vi "teste_corrente_2LEM.vi"() -> ()   [LabVIEW 2019]
uses:
  <vilib>/Analysis/5stat.llb/RMS (DBL).vi
  <vilib>/Analysis/NI_AALPro.lvlib
  <vilib>/Waveform/WDTFileIO.llb/ Write Waveforms to File (1D).vi
panel:
  in  "Nome de Base do Arquivo - Geral":string="medicoesGerais"
  out "Sucção [ºC]":dbl
  out "Reservatório [ºC]":dbl
  out "Descarga [ºC]":dbl
  out "Corpo [ºC]":dbl
  out "XY Graph 2":cluster{dbl[], dbl[]}[](graph)
  out "Corrente 2 RMS [A]":dbl
  out "Waveform Graph":dynamicdata(graph)
  out "Waveform Chart":dbl[][](graph)
  in  "stop":bool
  out "Corrente RMS [A]":dbl
  in  "Nome de Base do Arquivo - Corrente":string="corr"
  out "Erro Corrente":errorcluster
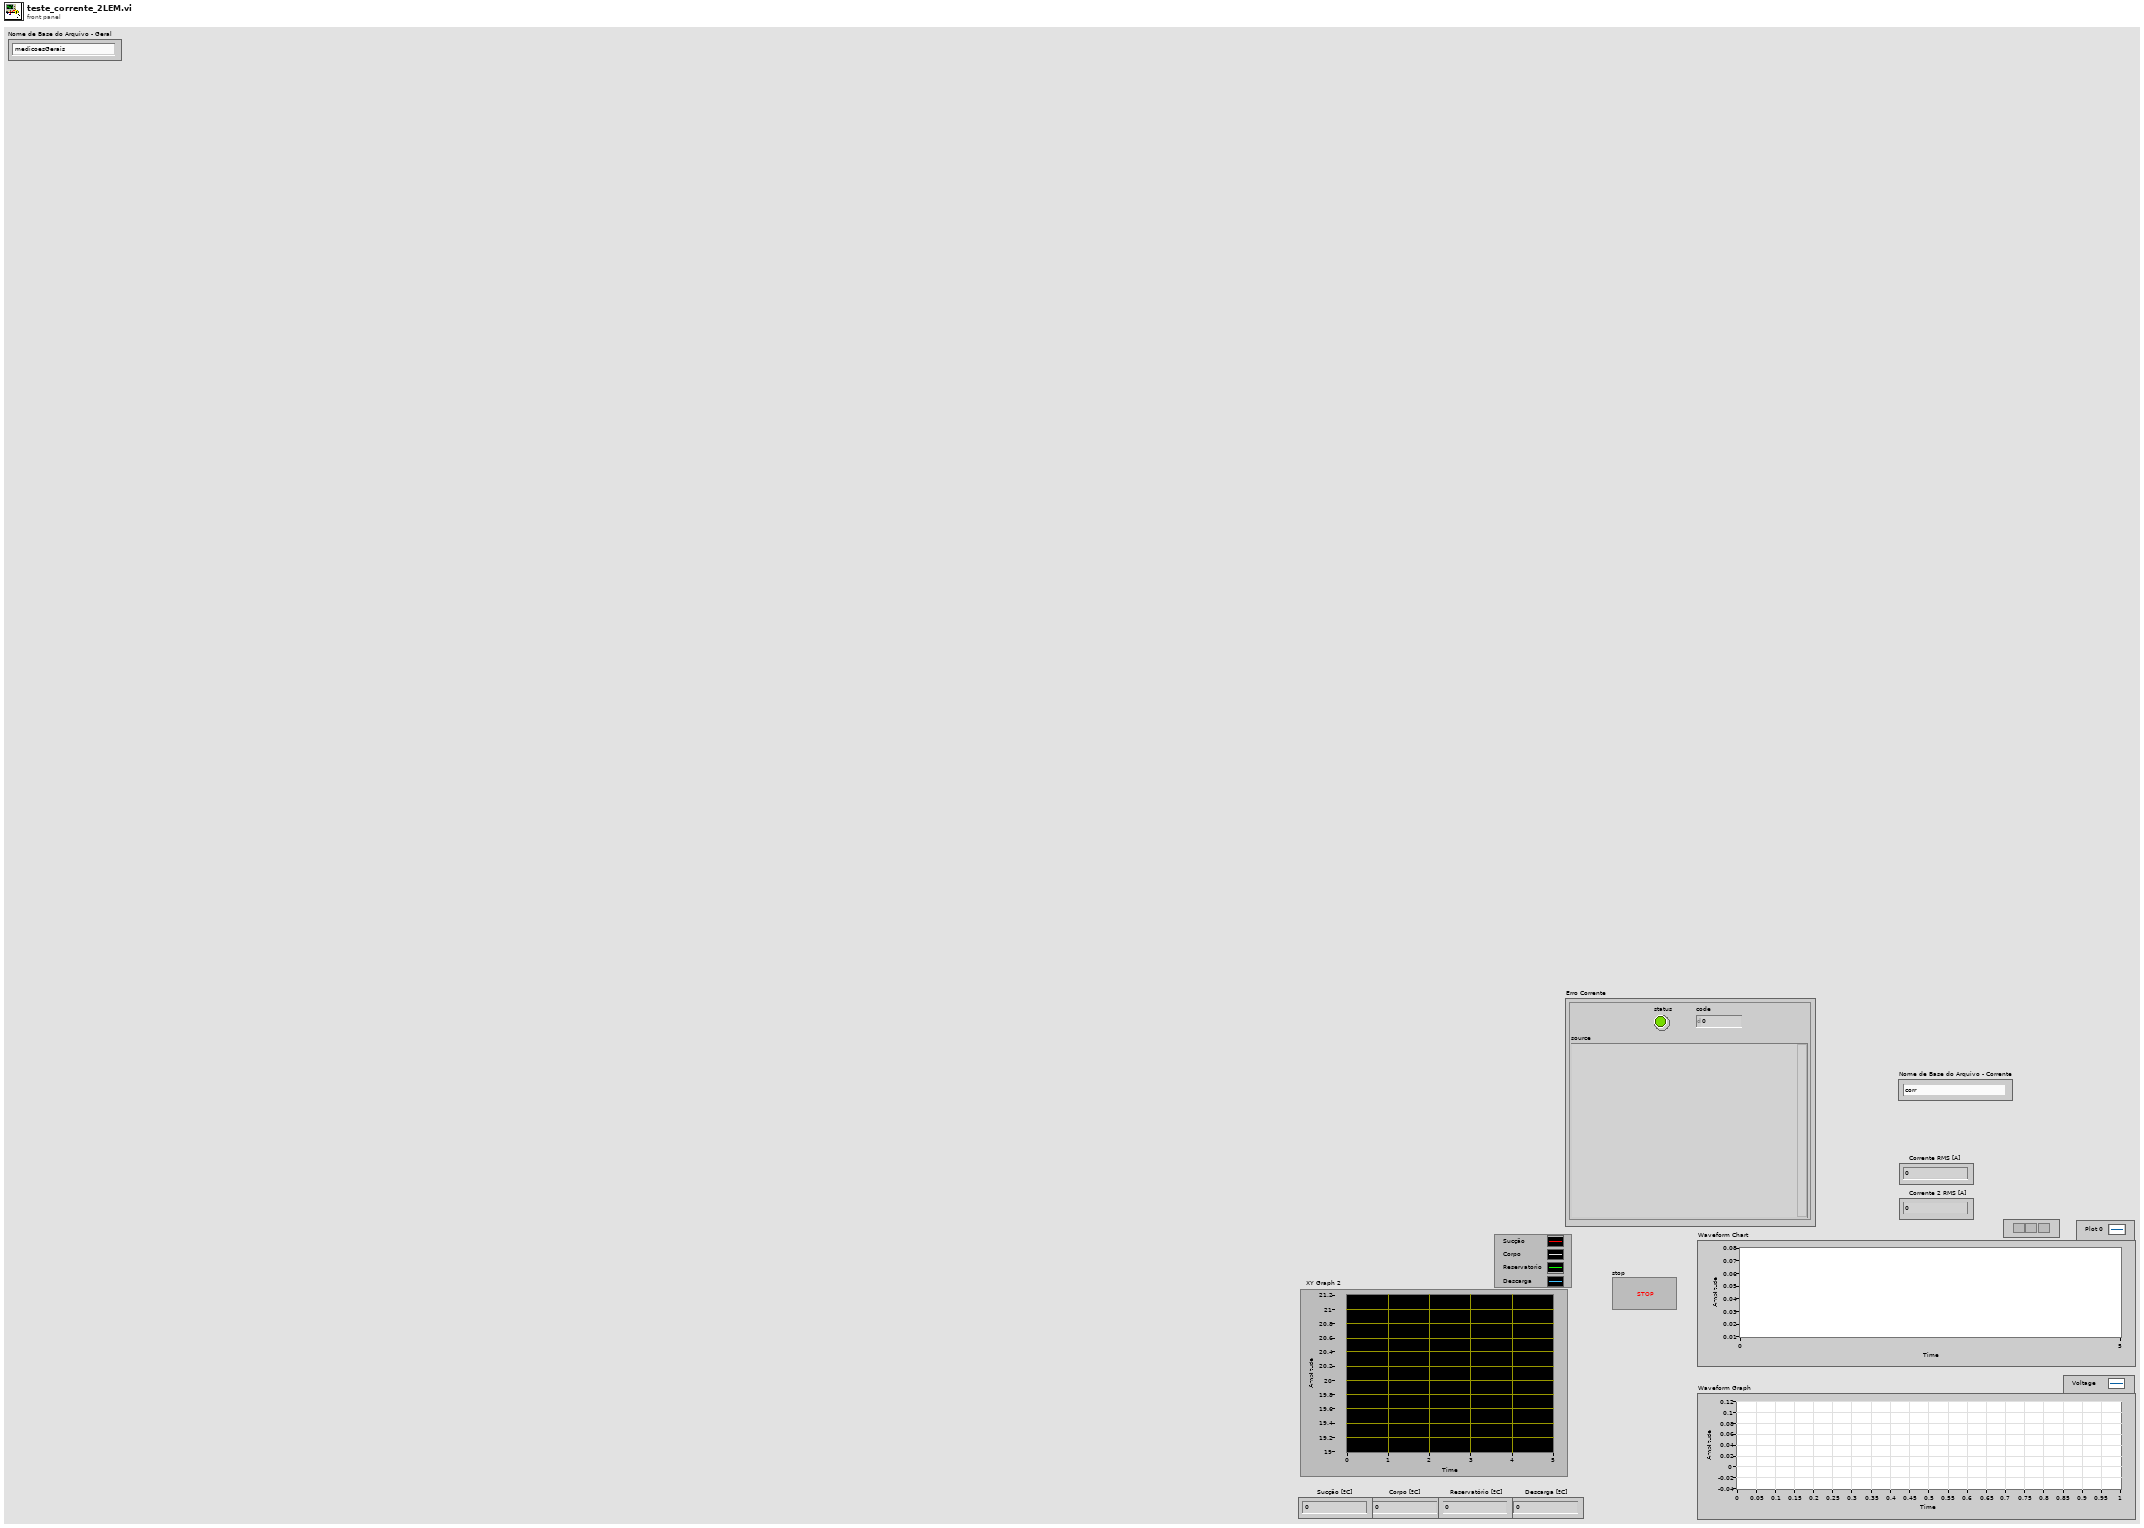
[diagram p1: front panel]
types:
  T1 = enum16{"open", "replace", "create", "open or create", "replace or create", "replace or create with confirmation"}
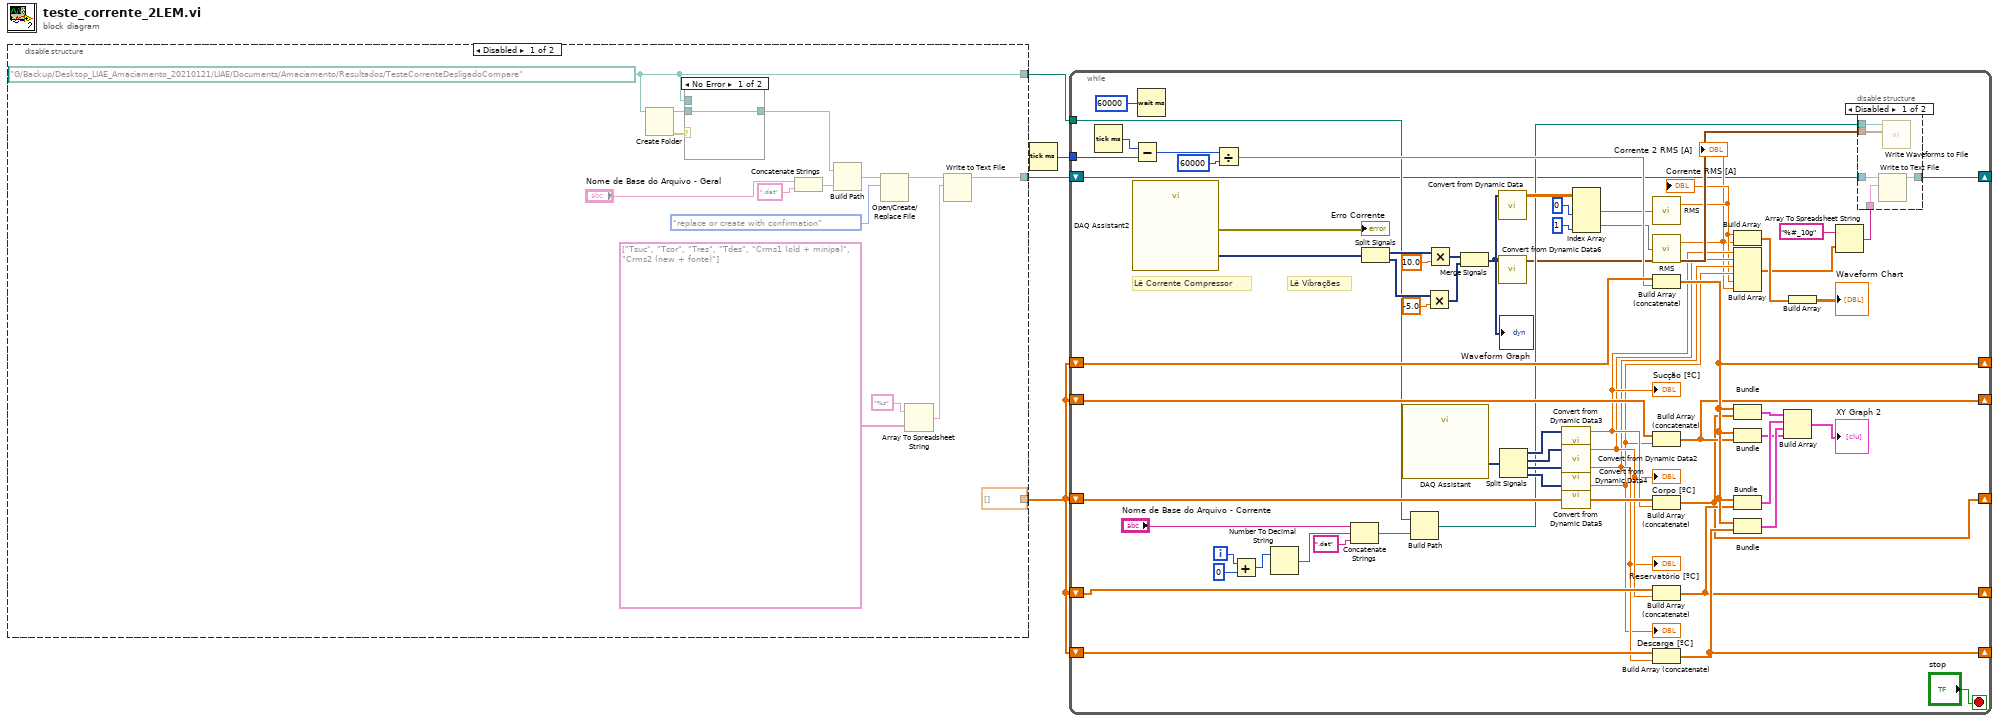
[diagram p0: block diagram]
diagram:
  n1 = disable-structure shown="Disabled" {
    disable-tunnel: [dbl[] [] _] -> w3
    disable-tunnel: [w6 _] -> w2
    disable-tunnel: [w5 _] -> w1
    frame Disabled {
      w5 = path "G:/Backup/Desktop_LIAE_Amaciamento_20210121/LIAE/Documents/Amaciamento/Resultados/TesteCorrenteDesligadoCompare" ("base path")
      n2 = Create Folder(path (use dialog)=w5) -> (created path=w10:path, error out=w11:errorcluster)  [unwired: 2 in, 1 out]
      n3 = case shown="No Error" w11 {
        tunnel: w10 -> [w20 _]
        tunnel: [w20 w21] -> w9
        tunnel: w5 -> [_ w21]
        frame No Error {
        }
        frame Error {
        }
      }
      n4 = Concatenate Strings("Nome de Base do Arquivo - Geral", ".dat") -> (w13:string)
      n5 = Build Path(base path=w9, name or relative path=w13) -> (appended path=w12:path)
      n6 = Open/Create/Replace File(file path (use dialog)=w12, operation (0:open)=T1."replace or create with confirmation") -> (refnum out=w17:refnum<file>)  [unwired: 4 in, 2 out]
      n7 = Array To Spreadsheet String(array=string[] ["Tsuc", "Tcor", "Tres", "Tdes", "Crms1 (old + minipa)", "Crms2 (new + fonte)"], 3:"%s" ("format string")) -> (spreadsheet string=w18:string)  [unwired: 1 in]
      n8 = Write to Text File(file (use dialog)=w17, text=w18) -> (refnum out=w6:refnum<file>)  [unwired: 2 in, 2 out]
    }
    frame Enabled {
    }
  }
  n9 = Tick Count (ms)() -> (millisecond timer value=w4:u32)
  n10 = while {
    tunnel: w4 -> [w78]
    shift-right: [w67] -> _
    shift-left: w3 -> [w66]
    shift-right: [w69] -> _
    shift-left: w3 -> [w68]
    shift-right: [w71] -> _
    shift-left: w3 -> [w70]
    shift-right: [w73] -> _
    shift-left: w3 -> [w72]
    shift-right: [w74] -> _
    shift-left: w3 -> [w76]
    tunnel: w1 -> [w34]
    shift-right: [w22] -> _
    shift-left: w2 -> [w23]
    i -> [w33]
    stop <- "stop" stop-if-true
    # "Lê Vibrações"
    # "Lê Corrente Compressor"
    n11 = Tick Count (ms)() -> (millisecond timer value=w79:u32)
    n12 = call "DAQ Assistant2"() -> ("data"=w36:dynamicdata, "error out"=→"Erro Corrente":errorcluster)  [unwired: 17 in, 1 out]
    n13 = Subtract(x=w79, y=w78) -> (x-y=w80:u32)
    n14 = Wait (ms)(milliseconds to wait=u32 60000) -> ()  [unwired: 1 out]
    n15 = Divide(x=w80, y=u32 60000) -> (x/y=w75:dbl)
    n16 = Add(x=w33, y=0) -> (x+y=w44:i32)
    n17 = Number To Decimal String(number=w44) -> (decimal integer string=w39:string)  [unwired: 1 in]
    n18 = Concatenate Strings("Nome de Base do Arquivo - Corrente", w39, ".dat" ("string")) -> (w40:string)
    n19 = Split Signals(w36) -> (w46:dynamicdata, w50:dynamicdata)  [unwired: 2 in]
    n20 = call "DAQ Assistant"() -> ("data"=w85:dynamicdata)  [unwired: 17 in, 2 out]
    n21 = Build Path(base path=w34, name or relative path=w40) -> (appended path=w42:path)
    n22 = Multiply(x=w50, y=-5.0) -> (x*y=w51:dynamicdata)
    n23 = Multiply(x=w46, y=10.0) -> (x*y=w48:dynamicdata)
    n24 = Merge Signals(w48, w51) -> (w52:dynamicdata)
    "Waveform Graph" <- w52
    n25 = call "Convert from Dynamic Data"("Dynamic Data Type"=w52) -> ("Array"=w53:dbl[][])  [unwired: 3 in]
    n26 = call "Convert from Dynamic Data6"("Dynamic Data Type"=w52) -> ("Array of Waveform"=w37:waveform(dbl)[])  [unwired: 3 in]
    n27 = Split Signals(w85) -> (w84:dynamicdata, w83:dynamicdata, w82:dynamicdata, w81:dynamicdata)  [unwired: 4 in]
    n28 = call "Convert from Dynamic Data3"("Dynamic Data Type"=w84) -> ("Scalar"=w29:dbl)  [unwired: 3 in]
    "Sucção [ºC]" <- w29
    n29 = call "Convert from Dynamic Data2"("Dynamic Data Type"=w83) -> ("Scalar"=w28:dbl)  [unwired: 3 in]
    "Corpo [ºC]" <- w28
    n30 = call "Convert from Dynamic Data4"("Dynamic Data Type"=w82) -> ("Scalar"=w27:dbl)  [unwired: 3 in]
    "Reservatório [ºC]" <- w27
    n31 = call "Convert from Dynamic Data5"("Dynamic Data Type"=w81) -> ("Scalar"=w26:dbl)  [unwired: 3 in]
    "Descarga [ºC]" <- w26
    n32 = Index Array(array=w53, index (col) #1=0 ("disabled index (col)"), index (col) #2=1 ("index (col)")) -> (element #1=w56:dbl[], element #2=w57:dbl[])  [unwired: 2 in]
    n33 = call-poly <vilib>:"RMS.vi"("X"=w56) -> ("rms value"=w25:dbl)  [unwired: 1 out]
    "Corrente RMS [A]" <- w25
    n34 = call-poly <vilib>:"RMS.vi"("X"=w57) -> ("rms value"=w24:dbl)  [unwired: 1 out]
    "Corrente 2 RMS [A]" <- w24
    n35 = Build Array (concatenate)(w76, w75) -> (w74:dbl[])
    n36 = Build Array (concatenate)(w72, w26) -> (w73:dbl[])
    n37 = Build Array (concatenate)(w66, w29) -> (w67:dbl[])
    n38 = Build Array (concatenate)(w68, w28) -> (w69:dbl[])
    n39 = Build Array (concatenate)(w70, w27) -> (w71:dbl[])
    n40 = Build Array(w25, w24) -> (w59:dbl[])
    n41 = Build Array(w29, w28, w27, w26, w25, w24) -> (w30:dbl[])
    n42 = Bundle(w74, w67) -> (w64:cluster{dbl[], dbl[]})  [unwired: 1 in]
    n43 = Bundle(w74, w73) -> (w61:cluster{dbl[], dbl[]})  [unwired: 1 in]
    n44 = Bundle(w74, w69) -> (w63:cluster{dbl[], dbl[]})  [unwired: 1 in]
    n45 = Bundle(w74, w71) -> (w62:cluster{dbl[], dbl[]})  [unwired: 1 in]
    n46 = Build Array(w64, w63, w62, w61) -> (→"XY Graph 2":cluster{dbl[], dbl[]}[])
    n47 = Build Array(w59) -> (→"Waveform Chart":dbl[][])
    n48 = Array To Spreadsheet String(array=w30, 3:"%#_10g" ("text")) -> (spreadsheet string=w31:string)  [unwired: 1 in]
    n49 = disable-structure shown="Disabled" {
      disable-tunnel: w42 -> [w90 _]
      disable-tunnel: w37 -> [w89 _]
      disable-tunnel: w31 -> [w88 _]
      disable-tunnel: w23 -> [w87 _]
      disable-tunnel: [w86 _] -> w22
      frame Disabled {
        n50 = Write to Text File(file (use dialog)=w87, text=w88) -> (refnum out=w86:refnum<file>)  [unwired: 2 in, 2 out]
        n51 = call-poly <vilib>:"Write Waveforms to File.vi"("waveform array"=w89, "file path (dialog if empty)"=w90) -> ()  [unwired: 8 in, 2 out]
      }
      frame Enabled {
      }
    }
  }
